vi "MovableROIFit.vi"(0 "input array":i16[][](array[numeric]), 1 "calibration data":dbl[](array[numeric]) format="%.2f", 3 "Fit band":T7 {"center freq" format="%.2f"; "stop freq" format="%.2f"; "start" format="%.2f"}, 4 "RF Info":T2, 5 "Sub-Band Filter":T1 {"threshold" format="%.2f"; "Fit band"."center freq" format="%.2f"; "Fit band"."stop freq" format="%.2f"; "Fit band"."low freq" format="%.2f"}, 6 "FFT size for":u16(ring) items=["next 2^n", "8", "16", "32", "64", "128", "256", "512"], 7 "Fit array":T6, 8 "Proc Method":i32, 10 "freq (MHz)":dbl format="%.2f", 11 "Single ROI?":bool, 12 "subtract spectrum\nfrom fit?":bool, 13 "convert output to dB?":bool=TRUE) -> (9 "Freq Values":dbl[](array[numeric]), 14 "Raw Fit Data":T5 {"pts in fit" format="%.2f"; "midband fit" format="%.2f"; "intercept (b)" format="%.2f"; "slope (m)" format="%.2f"}, 15 "Cal params":T4 {"MSE" format="%.2f"; "pts in fit" format="%.2f"; "midband fit" format="%.2f"; "b stand dev" format="%.2f"; "intercept (b)" format="%.2f"; "m stand dev" format="%.2f"; "slope (m)" format="%.2f"}, 16 "STFT Sum":dbl[][](array[numeric]), 17 "Length of padded array":i32, 18 "Plots":T3(array[cluster]) {"?" format="%.2f"; "df (MHz)" format="%.2f"; "fo of fit" format="%.2f"}, 19 "power spectrum in dB":dbl[](array[numeric]) format="%.2f")   [LabVIEW 2022 SP3]
uses:
  <vilib>/Analysis/baseanly.llb/Mean (DBL).vi
  <vilib>/Analysis/baseanly.llb/Unit Vector (DBL).vi
  <vilib>/Analysis/4window.llb/Hamming Window (DBL).vi
  <vilib>/Analysis/2dsp.llb/Real FFT.vi
  <vilib>/Analysis/4window.llb/AllCosWindow (DBL).vi
  <vilib>/Analysis/0measdsp.llb/Scaled Time Domain Window (DBL).vi
  <vilib>/gmath/NI_Gmath.lvlib
  <vilib>/Analysis/NI_AALPro.lvlib
  <vilib>/Analysis/NI_AALBase.lvlib
panel:
  out "Cal File Att":dbl format="%.2f"
  out "RF File Att":dbl format="%.2f"
  # "Spectrum Fit Parameters"
  # "`"
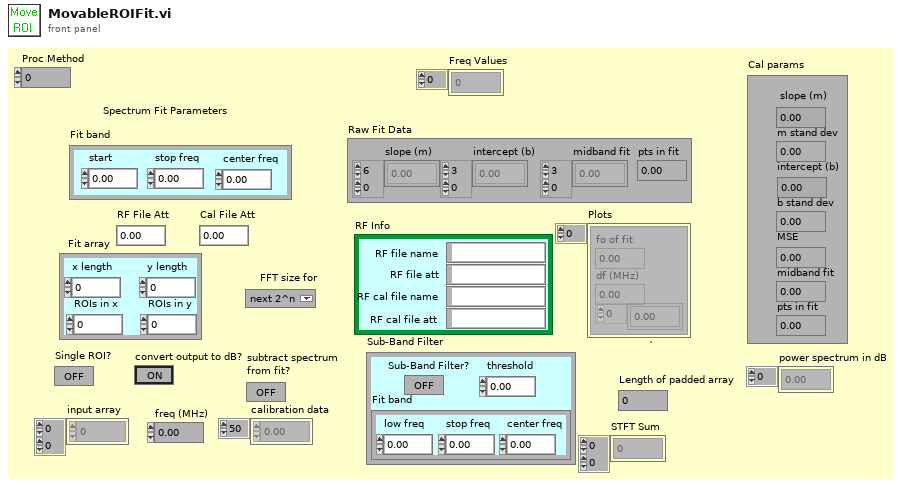
[diagram p1: front panel]
types:
  T1 = cluster{"Fit band":cluster{"low freq":dbl, "stop freq":dbl, "center freq":dbl}, "threshold":dbl, "Sub-Band Filter?":bool}
  T2 = cluster{"RF file name":string, "RF file att":string, "RF cal file name":string, "RF cal file att":string}
  T3 = cluster{"fo of fit":dbl, "df (MHz)":dbl, dbl[]}[]
  T4 = cluster{"slope (m)":dbl, "m stand dev":dbl, "intercept (b)":dbl, "b stand dev":dbl, "MSE":dbl, "midband fit":dbl, "pts in fit":dbl}
  T5 = cluster{"slope (m)":dbl[][], "intercept (b)":dbl[][], "midband fit":dbl[][], "pts in fit":dbl}
  T6 = cluster{"x length":i32, "y length":i32, "ROIs in x":i32, "ROIs in y":i32}
  T7 = cluster{"start":dbl, "stop freq":dbl, "center freq":dbl}
  T8 = cluster{"low freq":dbl, "stop freq":dbl, "center freq":dbl}
  T9 = cluster{"force freq bins to power of 2?":bool, "exclude Nyquist frequency?":bool}
  T10 = cluster{dbl, "x length":i32, dbl, "y length":i32}
  T11 = cluster{"x length":dbl, "x length":i32, "ROIs in x":dbl, "y length":i32}
  T12 = cluster{dbl[][], dbl[][], dbl[][], "pts in fit":dbl}
  T13 = cluster{i32, dbl, "power spectrum in dB":dbl[]}[]
  T14 = cluster{"fo of fit":dbl, dbl, "power spectrum in dB":dbl[]}[]
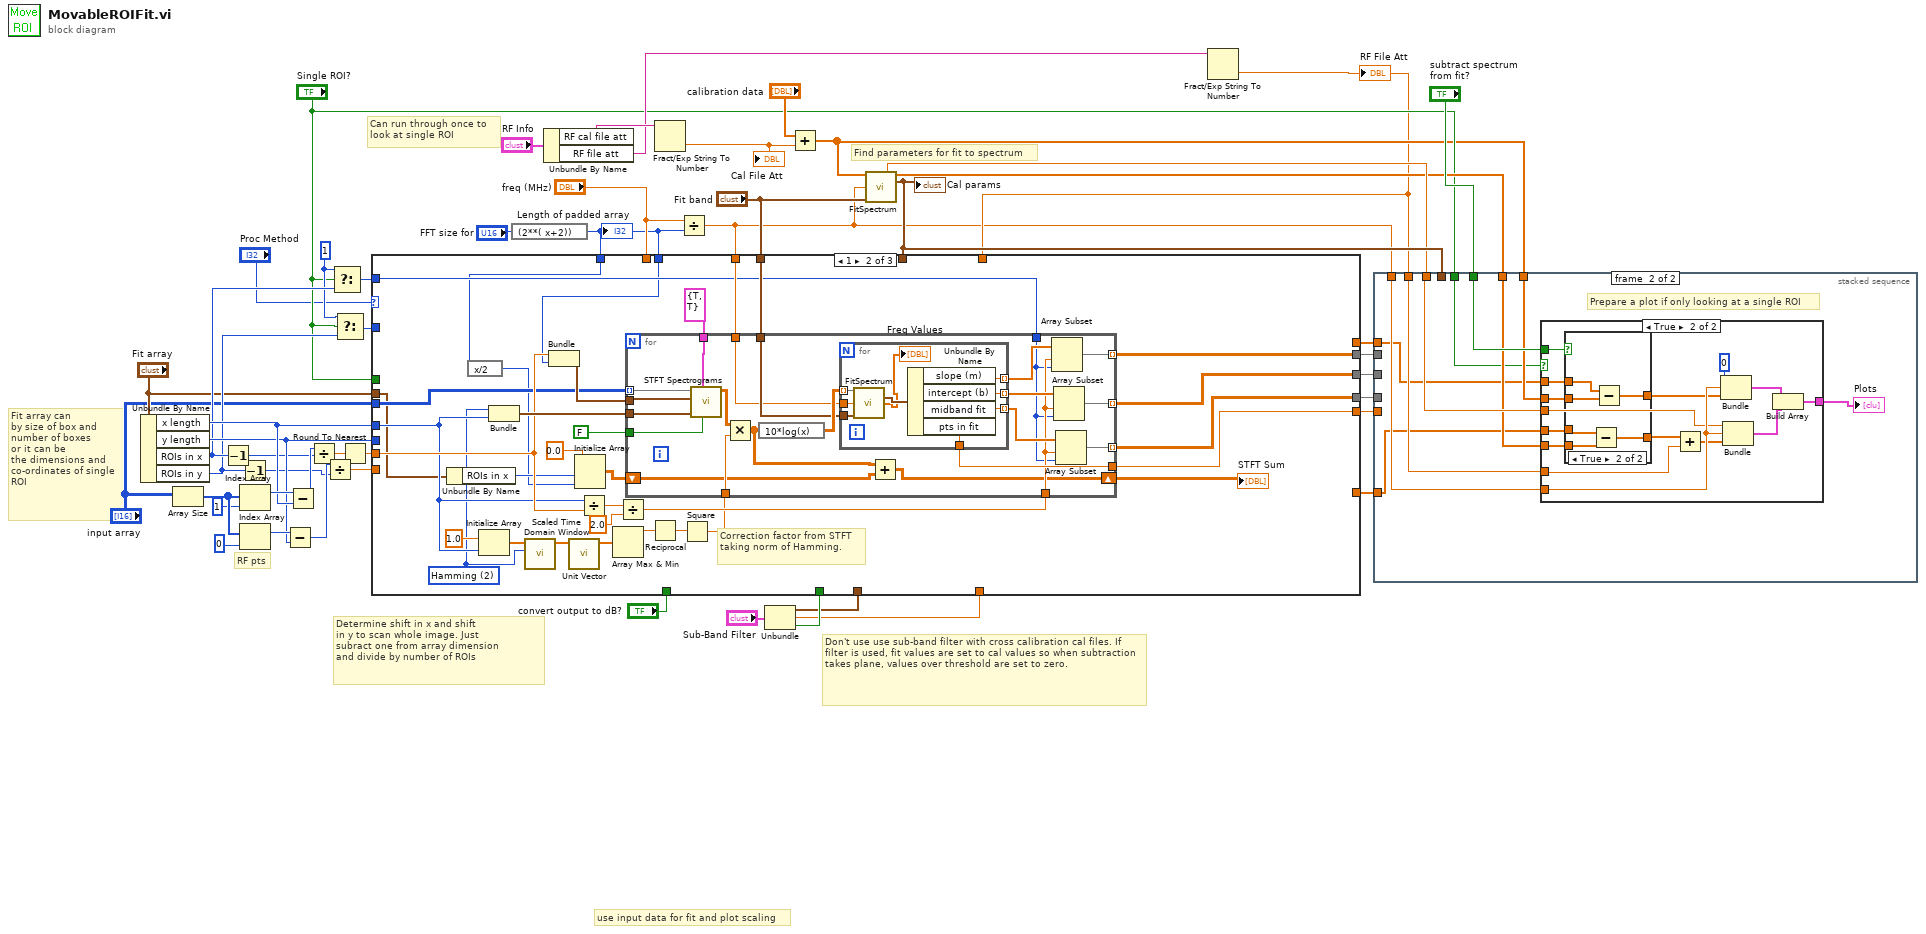
[diagram p0: block diagram]
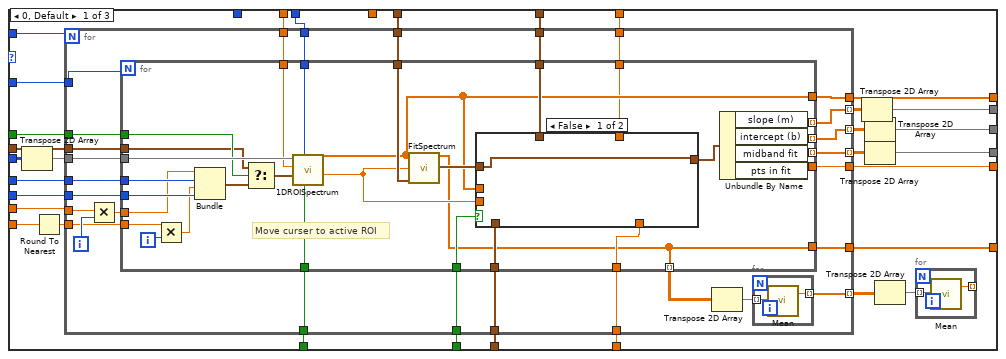
[diagram p2: hidden frame]
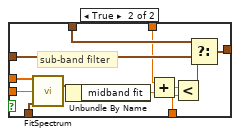
[diagram p3: hidden frame]
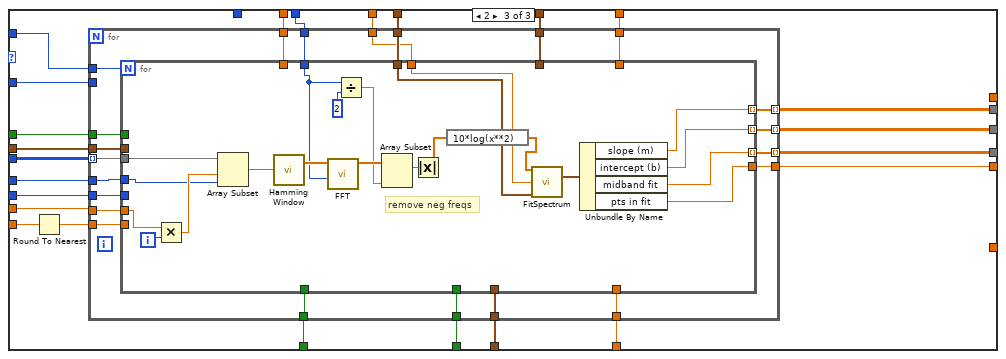
[diagram p4: hidden frame]
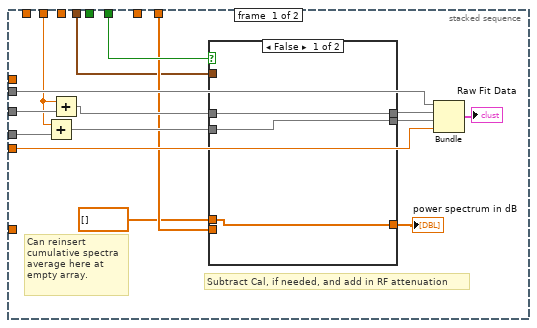
[diagram p5: hidden frame]
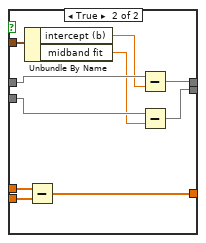
[diagram p6: hidden frame]
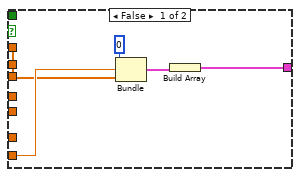
[diagram p7: hidden frame]
diagram:
  w33 = 1 ("t")
  # "RF pts"
  # "Don't use use sub-band filter with cross calibration cal files. If filter is used, fit values are set to cal values so when subtraction takes plane, values over threshold are set to zero."
  # "Determine shift in x and shift\nin y to scan whole image. Just\nsubract one from array dimension\nand divide by number of ROIs"
  # "Can run through once to\nlook at single ROI"
  # "Find parameters for fit to spectrum"
  # "Fit array can\nby size of box and \nnumber of boxes\nor it can be\nthe dimensions and\nco-ordinates of single\nROI"
  # "use input data for fit and plot scaling"
  n1 = Unbundle By Name("Fit array") -> ("x length"=w43:i32, "y length"=w42:i32, "ROIs in x"=w36:i32, "ROIs in y"=w34:i32)
  n2 = Array Size(array="input array") -> (size(s)=w50:i32[])
  n3 = Decrement(x=w36) -> (x-1=w40:i32)
  n4 = Decrement(x=w34) -> (x-1=w39:i32)
  n5 = Index Array(array=w50, index=1 ("Index")) -> (element=w46:i32)
  n6 = Index Array(array=w50, index=0 ("Index")) -> (element=w44:i32)
  n7 = Subtract(x=w44, y=w42) -> (x-y=w45:i32)
  n8 = Subtract(x=w46, y=w43) -> (x-y=w41:i32)
  n9 = Divide(x=w41, y=w40) -> (x/y=w14:dbl)
  n10 = Divide(x=w45, y=w39) -> (x/y=w5:dbl)
  n11 = Select(t=w33, s="Single ROI?", f=w36) -> (s? t:f=w3:i32)
  n12 = Select(t=w33, s="Single ROI?", f=w34) -> (s? t:f=w35:i32)
  n13 = Round To Nearest(number=w14) -> (nearest integer value=w15:dbl)
  n14 = expression code="(2**( x+2))"("FFT size for") -> (w1:u16)
  "Length of padded array" <- w1
  n15 = Unbundle By Name("RF Info") -> ("RF cal file att"=w29:string, "RF file att"=w28:string)
  n16 = Fract/Exp String To Number(string=w29) -> (number=w27:dbl)  [unwired: 4 out]
  "Cal File Att" <- w27
  n17 = Divide(x="freq (MHz)", y=w1) -> (x/y=w6:dbl)
  n18 = Unbundle("Sub-Band Filter") -> ("Fit band"=w24:T8, "threshold"=w23:dbl, "Sub-Band Filter?"=w25:bool)
  n19 = Add(x="calibration data", y=w27) -> (x+y=w8:dbl[])
  n20 = call "FitSpectrum.vi"("Y Values"=w8, "df (MHz)"=w6, "Fit band"="Fit band") -> ("fo of fit"=w12:dbl, "Best Linear Fit"=w11:dbl[], "Cluster"=w16:T4)  [unwired: 10 out]
  "Cal params" <- w16
  n21 = Fract/Exp String To Number(string=w28) -> (number=w7:dbl)  [unwired: 4 out]
  "RF File Att" <- w7
  n22 = case shown="1" "Proc Method" {
    tunnel: [w81 w184 w243] -> w47
    tunnel: w43 -> [w80 w174 w242]
    tunnel: w42 -> [w79 _ w241]
    tunnel: "Fit band" -> [w78 w188 w240]
    tunnel: "convert output to dB?" -> [w77 _ w239]
    tunnel: w3 -> [w76 w179 w224]
    tunnel: w35 -> [w75 _ w238]
    tunnel: "Fit array" -> [w74 w159 w237]
    tunnel: w25 -> [w73 _ w236]
    tunnel: w24 -> [w72 _ w235]
    tunnel: w23 -> [w71 _ w234]
    tunnel: "freq (MHz)" -> [w70 _ w233]
    tunnel: w1 -> [w69 w177 w232]
    tunnel: [w54 w164 w222] -> w20
    tunnel: [w53 w165 w221] -> w19
    tunnel: [w55 w163 w223] -> w18
    tunnel: w16 -> [w68 _ w231]
    tunnel: w15 -> [w67 w183 w230]
    tunnel: [w65 _ _] -> w13
    tunnel: [w64 _ _] -> w10
    tunnel: "Single ROI?" -> [w63 _ w228]
    tunnel: w7 -> [w62 _ w227]
    tunnel: "input array" -> [w60 w167 w220]
    tunnel: w5 -> [w61 _ w226]
    tunnel: w6 -> [_ w187 w225]
    tunnel: w1 -> [_ w157 _]
    frame 0, Default {
      n23 = Transpose 2D Array(2D array=w60) -> (transposed array=w59:i16[][])
      n24 = Round To Nearest(number=w61) -> (nearest integer value=w66:dbl)
      n25 = for {
        N: w76 -> [_]
        tunnel: w69 -> [w111]
        tunnel: w59 -> [w110]
        tunnel: w80 -> [w109]
        tunnel: w79 -> [w108]
        tunnel: w75 -> [w107]
        tunnel: w78 -> [w106]
        tunnel: w67 -> [w104]
        tunnel: w66 -> [w102]
        tunnel: [w101] -> w58 mode=indexing
        tunnel: [w100] -> w57 mode=indexing
        tunnel: [w99] -> w56 mode=indexing
        tunnel: [w98] -> w81
        tunnel: w70 -> [w97]
        tunnel: [w96] -> w64
        tunnel: w74 -> [w95]
        tunnel: w63 -> [w94]
        tunnel: w77 -> [w93]
        tunnel: w73 -> [w92]
        tunnel: w72 -> [w91]
        tunnel: w71 -> [w90]
        tunnel: [w89] -> w65
        tunnel: w68 -> [w88]
        tunnel: w62 -> [w87]
        tunnel: [w84] -> w51 mode=indexing
        i -> [w105]
        n26 = Multiply(x=w104, y=w105) -> (x*y=w103:dbl)
        n27 = for {
          N: w107 -> [_]
          tunnel: w111 -> [w142]
          tunnel: w110 -> [w139]
          tunnel: w109 -> [w127]
          tunnel: w108 -> [w126]
          tunnel: w106 -> [w133]
          tunnel: w103 -> [w118]
          tunnel: w102 -> [w140]
          tunnel: [w138] -> w101 mode=indexing
          tunnel: [w137] -> w100 mode=indexing
          tunnel: [w136] -> w99 mode=indexing
          tunnel: [w135] -> w98
          tunnel: w97 -> [w134]
          tunnel: [w114] -> w96
          tunnel: w95 -> [w128]
          tunnel: w94 -> [w129]
          tunnel: w93 -> [w130]
          tunnel: w92 -> [w125]
          tunnel: w91 -> [w123]
          tunnel: w90 -> [w116]
          tunnel: w88 -> [w120]
          tunnel: [w119] -> w89
          tunnel: w87 -> [w115]
          tunnel: [w114] -> w86 mode=indexing
          i -> [w141]
          # "Move curser to active ROI"
          n28 = Multiply(x=w140, y=w141) -> (x*y=w117:dbl)
          n29 = Bundle(w118, "x length"=w127, w117, "y length"=w126) -> (w131:T10)  [unwired: 1 out]
          n30 = Select(t=w128, s=w129, f=w131) -> (s? t:f=w132:T11)
          n31 = call "1DROISpectrum.vi"("convert output to dB?"=w130, "Length of padded array"=w142, "Array Subset"=w132, "freq (MHz)"=w134, "2-D data array"=w139) -> ("df (MHz)"=w124:dbl, "power spectrum in dB"=w119:dbl[])  [unwired: 5 out]
          n32 = call "FitSpectrum.vi"("Y Values"=w119, "df (MHz)"=w124, "Fit band"=w133) -> ("Best Linear Fit"=w114:dbl[], "Cluster"=w122:T4)  [unwired: 11 out]
          n33 = case shown="False" w125 {
            tunnel: w124 -> [_ w155]
            tunnel: w123 -> [_ w154]
            tunnel: w116 -> [_ w152]
            tunnel: w122 -> [w143 w148]
            tunnel: [w143 w150] -> w121
            tunnel: w120 -> [_ w149]
            tunnel: w119 -> [_ w147]
            tunnel: w115 -> [_ w145]
            frame False {
            }
            frame True {
              # "sub-band filter"
              n34 = call "FitSpectrum.vi"("Y Values"=w147, "df (MHz)"=w155, "Fit band"=w154) -> ("Cluster"=w153:T4)  [unwired: 12 out]
              n35 = Unbundle By Name(w153) -> ("midband fit"=w146:dbl)
              n36 = Add(x=w145, y=w146) -> (x+y=w144:dbl)
              n37 = Less?(x=w144, y=w152) -> (x < y?=w151:bool)
              n38 = Select(t=w149, s=w151, f=w148) -> (s? t:f=w150:T4)
            }
          }
          n39 = Unbundle By Name(w121) -> ("slope (m)"=w138:dbl, "intercept (b)"=w137:dbl, "midband fit"=w136:dbl, "pts in fit"=w135:dbl)
        }
        n40 = Transpose 2D Array(2D array=w86) -> (transposed array=w85:dbl[][])
        n41 = for {
          tunnel: w85 -> [w113] mode=indexing
          tunnel: [w112] -> w84 mode=indexing
          n42 = call-poly <vilib>:"Mean.vi"("X"=w113) -> ("mean"=w112:dbl)  [unwired: 1 out]
        }
      }
      n43 = Transpose 2D Array(2D array=w58) -> (transposed array=w55:dbl[][])
      n44 = Transpose 2D Array(2D array=w57) -> (transposed array=w54:dbl[][])
      n45 = Transpose 2D Array(2D array=w56) -> (transposed array=w53:dbl[][])
      n46 = Transpose 2D Array(2D array=w51) -> (transposed array=w52:dbl[][])
      n47 = for {
        tunnel: w52 -> [w83] mode=indexing
        tunnel: [w82] -> _ mode=indexing
        n48 = call-poly <vilib>:"Mean.vi"("X"=w83) -> ("mean"=w82:dbl)  [unwired: 1 out]
      }
    }
    frame 1 {
      w173 = u32 2 items=["Rectangle"=0, "Hanning"=1, "Hamming"=2, "Blackman-Harris"=3, "Exact Blackman"=4, "Blackman"=5, "Flat Top"=6, "4 Term B-Harris "=7, "7 Term B-Harris"=8, "Low Sidelobe"=9, "Blackman Nuttall"=11, "Triangle"=30, "Gaussian"=62] ("type")
      # "Correction factor from STFT taking norm of Hamming."
      n49 = Unbundle By Name(w159) -> ("ROIs in x"=w158:i32)
      n50 = expression code="x/2"(w157) -> (w156:u16)
      n51 = Initialize Array(1.0 ("element"), w174) -> (w175:dbl[])
      n52 = Bundle("type"=w173, "x length"=w174) -> (w185:cluster{"type":u32, "x length":i32})  [unwired: 1 in]
      n53 = call-poly <vilib>:"Scaled Time Domain Window.vi"("window"=w173, "X"=w175) -> ("Windowed X"=w172:dbl[])  [unwired: 7 in, 2 out]
      n54 = Bundle(w183, "FFT size for"=w177) -> (w186:cluster{dbl, "FFT size for":u16})  [unwired: 1 in]
      n55 = call-poly <vilib>:"Unit Vector.vi"("Input Vector"=w172) -> ("Unit Vector"=w171:dbl[])  [unwired: 8 in, 2 out]
      n56 = Initialize Array(0.0, w158, w156) -> (w160:dbl[][])
      n57 = Divide(x=w174, y=w183) -> (x/y=w182:dbl)
      n58 = Array Max & Min(array=w171) -> (max value=w169:dbl)  [unwired: 3 out]
      n59 = Divide(x=w182, y=2.0) -> (x/y=w180:dbl)
      n60 = Reciprocal(x=w169) -> (1/x=w168:dbl)
      n61 = Square(x=w168) -> (x^2=w170:dbl)
      n62 = for {
        tunnel: w188 -> [w209]
        tunnel: w187 -> [w208]
        tunnel: w186 -> [w207]
        tunnel: w185 -> [w206]
        tunnel: [w202] -> w163 mode=indexing
        tunnel: [w200] -> w164 mode=indexing
        tunnel: [w199] -> w165 mode=indexing
        tunnel: [w205] -> w184
        tunnel: w167 -> [w204] mode=indexing
        tunnel: w180 -> [w197]
        tunnel: w179 -> [w196]
        tunnel: FALSE ("energy conservation?") -> [w195]
        tunnel: w170 -> [w193]
        tunnel: T9 {"force freq bins to power of 2?"=TRUE, "exclude Nyquist frequency?"=TRUE} ("time-freq config") -> [w192]
        shift-right: [w190] -> w162
        shift-left: w160 -> [w189]
        n63 = call <vilib>:"STFT Spectrograms.vi"("energy conservation?"=w195, "time-freq config"=w192, "window info"=w206, "time-freq sampling info"=w207, "X"=w204) -> ("STFT Spectrogram {X}"=w194:dbl[][])  [unwired: 5 in, 1 out]
        n64 = Multiply(x=w194, y=w193) -> (x*y=w191:dbl[][])
        n65 = expression code="10*log(x)"(w191) -> (w210:dbl[][])
        n66 = for {
          tunnel: w210 -> [w219] mode=indexing
          tunnel: [w217] -> w203 mode=indexing
          tunnel: [w216] -> w201 mode=indexing
          tunnel: [w215] -> w198 mode=indexing
          tunnel: [w214] -> w205
          tunnel: w209 -> [w213]
          tunnel: w208 -> [w212]
          n67 = call "FitSpectrum.vi"("Y Values"=w219, "df (MHz)"=w212, "Fit band"=w213) -> ("Cluster"=w218:T4, "Freq Values"=→"Freq Values":dbl[])  [unwired: 11 out]
          n68 = Unbundle By Name(w218) -> ("slope (m)"=w217:dbl, "intercept (b)"=w216:dbl, "midband fit"=w215:dbl, "pts in fit"=w214:dbl)
        }
        n69 = Add(x=w191, y=w189) -> (x+y=w190:dbl[][])
        n70 = Array Subset(array=w203, index=w197, length=w196) -> (w202:dbl[])
        n71 = Array Subset(array=w201, index=w197, length=w196) -> (w200:dbl[])
        n72 = Array Subset(array=w198, index=w197, length=w196) -> (w199:dbl[])
      }
      "STFT Sum" <- w162
    }
    frame 2 {
      n73 = Round To Nearest(number=w226) -> (nearest integer value=w229:dbl)
      n74 = for {
        tunnel: w232 -> [w265]
        tunnel: w220 -> [w264] mode=indexing
        tunnel: w242 -> [w263]
        tunnel: w241 -> [w262]
        tunnel: w238 -> [_]
        tunnel: w240 -> [w261]
        tunnel: w230 -> [w244]
        tunnel: w229 -> [w260]
        tunnel: [w259] -> w223 mode=indexing
        tunnel: [w258] -> w222 mode=indexing
        tunnel: [w257] -> w221 mode=indexing
        tunnel: [w256] -> w243
        tunnel: w233 -> [w255]
        tunnel: w237 -> [w254]
        tunnel: w228 -> [w253]
        tunnel: w239 -> [w252]
        tunnel: w236 -> [w251]
        tunnel: w235 -> [w250]
        tunnel: w234 -> [w249]
        tunnel: w231 -> [w248]
        tunnel: w227 -> [w247]
        tunnel: w225 -> [w246]
        tunnel: w224 -> [w245]
        n75 = for {
          N: w245 -> [_]
          tunnel: w265 -> [w278]
          tunnel: w264 -> [w280]
          tunnel: w263 -> [w281]
          tunnel: w262 -> [_]
          tunnel: w261 -> [w274]
          tunnel: w260 -> [_]
          tunnel: [w272] -> w259 mode=indexing
          tunnel: [w271] -> w258 mode=indexing
          tunnel: [w270] -> w257 mode=indexing
          tunnel: [w269] -> w256
          tunnel: w255 -> [_]
          tunnel: w254 -> [_]
          tunnel: w253 -> [_]
          tunnel: w252 -> [_]
          tunnel: w251 -> [_]
          tunnel: w250 -> [_]
          tunnel: w249 -> [_]
          tunnel: w248 -> [_]
          tunnel: w247 -> [_]
          tunnel: w246 -> [w275]
          tunnel: w244 -> [w268]
          i -> [w286]
          # "remove neg freqs"
          n76 = Multiply(x=w268, y=w286) -> (x*y=w282:dbl)
          n77 = Array Subset(array=w280, index=w282, length=w281) -> (w279:i16[])
          n78 = call-poly <vilib>:"Hamming Window.vi"("X"=w279) -> ("Windowed X"=w283:dbl[])  [unwired: 1 out]
          n79 = call-poly <vilib>:"FFT.vi"("FFT size"=w278, "X"=w283) -> ("FFT {X}"=w284:cdb[])  [unwired: 1 in, 8 out]
          n80 = Divide(x=w278, y=2) -> (x/y=w277:dbl)
          n81 = Array Subset(array=w284, length=w277) -> (w276:cdb[])  [unwired: 1 in]
          n82 = Absolute Value(x=w276) -> (abs(x)=w267:dbl[])
          n83 = expression code="10*log(x**2)"(w267) -> (w266:dbl[])
          n84 = call "FitSpectrum.vi"("Y Values"=w266, "df (MHz)"=w275, "Fit band"=w274) -> ("Cluster"=w273:T4)  [unwired: 12 out]
          n85 = Unbundle By Name(w273) -> ("slope (m)"=w272:dbl, "intercept (b)"=w271:dbl, "midband fit"=w270:dbl, "pts in fit"=w269:dbl)
        }
      }
    }
  }
  n86 = stacked-sequence {
    tunnel: w47 -> [w301 _]
    tunnel: w20 -> [w300 _]
    tunnel: w19 -> [w299 _]
    tunnel: w18 -> [w297 _]
    tunnel: "subtract spectrum\nfrom fit?" -> [w292 w323]
    tunnel: w7 -> [w291 w324]
    tunnel: w8 -> [w289 w322]
    tunnel: w16 -> [w288 _]
    tunnel: w13 -> [_ w316]
    tunnel: w12 -> [_ w321]
    tunnel: w11 -> [_ w320]
    tunnel: w10 -> [_ w315]
    tunnel: w6 -> [_ w319]
    tunnel: "Single ROI?" -> [_ w317]
    frame #0 {
      # "Subtract Cal, if needed, and add in RF attenuation"
      # "Can reinsert cumulative spectra average here at empty array."
      n87 = Add(x=w291, y=w299) -> (x+y=w296:dbl[][])
      n88 = Add(x=w291, y=w300) -> (x+y=w295:dbl[][])
      n89 = case shown="False" w292 {
        tunnel: [w304 w314] -> w298
        tunnel: dbl[] [] -> [w304 w313]
        tunnel: w289 -> [_ w312]
        tunnel: [w302 w306] -> w294
        tunnel: w296 -> [w302 w310]
        tunnel: [w303 w307] -> w293
        tunnel: w295 -> [w303 w311]
        tunnel: w288 -> [_ w305]
        frame False {
        }
        frame True {
          n90 = Unbundle By Name(w305) -> ("intercept (b)"=w309:dbl, "midband fit"=w308:dbl)
          n91 = Subtract(x=w313, y=w312) -> (x-y=w314:dbl[])
          n92 = Subtract(x=w311, y=w309) -> (x-y=w307:dbl[][])
          n93 = Subtract(x=w310, y=w308) -> (x-y=w306:dbl[][])
        }
      }
      "power spectrum in dB" <- w298
      n94 = Bundle(w297, w293, w294, "pts in fit"=w301) -> (→"Raw Fit Data":T12)  [unwired: 1 out]
    }
    frame #1 {
      # "Prepare a plot if only looking at a single ROI"
      n95 = case shown="True" w317 {
        tunnel: w320 -> [_ w342]
        tunnel: w322 -> [_ w333]
        tunnel: w315 -> [_ w338]
        tunnel: w319 -> [w327 w341]
        tunnel: w321 -> [_ w340]
        tunnel: [w326 w337] -> w318
        tunnel: w323 -> [_ w336]
        tunnel: w316 -> [w325 w335]
        tunnel: w324 -> [_ w330]
        frame False {
          n96 = Bundle(0, w327, "power spectrum in dB"=w325) -> (w328:cluster{i32, dbl, "power spectrum in dB":dbl[]})  [unwired: 1 out]
          n97 = Build Array(w328) -> (w326:T13)
        }
        frame True {
          n98 = case shown="True" w336 {
            tunnel: w342 -> [_ w352]
            tunnel: [w346 w350] -> w332
            tunnel: w338 -> [w346 w351]
            tunnel: w335 -> [w345 w349]
            tunnel: [w345 w348] -> w334
            tunnel: w333 -> [_ w347]
            frame False {
            }
            frame True {
              n99 = Subtract(x=w351, y=w352) -> (x-y=w350:dbl[])
              n100 = Subtract(x=w349, y=w347) -> (x-y=w348:dbl[])
            }
          }
          n101 = Add(x=w332, y=w330) -> (x+y=w331:dbl[])
          n102 = Bundle(0, w341, "power spectrum in dB"=w334) -> (w343:cluster{i32, dbl, "power spectrum in dB":dbl[]})  [unwired: 1 out]
          n103 = Bundle("fo of fit"=w340, w341, w331) -> (w339:cluster{"fo of fit":dbl, dbl, dbl[]})  [unwired: 1 out]
          n104 = Build Array(w343, w339) -> (w337:T14)
        }
      }
      "Plots" <- w318
    }
  }
